vi "AdaptToInputs.vi"(3 "Term Types":T1, 4 "XRef":refnum<vi>, 5 "State In":T5) -> (0 "Reply":string[](array[string]), 2 "State Out":T5)   [LabVIEW 2012, in "Array Size and Index.xnode"]
uses:
  Array Size and Index.xnode
  State.ctl
  <vilib>/XNodeSupport/XNodeTermTypeIDPairs.ctl
  <vilib>/XNodeSupport/XNodeTermTypeIDPair.ctl
  <vilib>/XNodeSupport/XNodeType.ctl
  <vilib>/XNodeSupport/XNodeString.ctl
  <userlib>/_LAVAcr/Scripting Tools/XNode Support/Find term type by ID_type.vi
  <userlib>/_LAVAcr/Scripting Tools/XNode Support/XNode Support.lvlib
  <vilib>/XNodeSupport/NI_XNodeSupport.lvlib
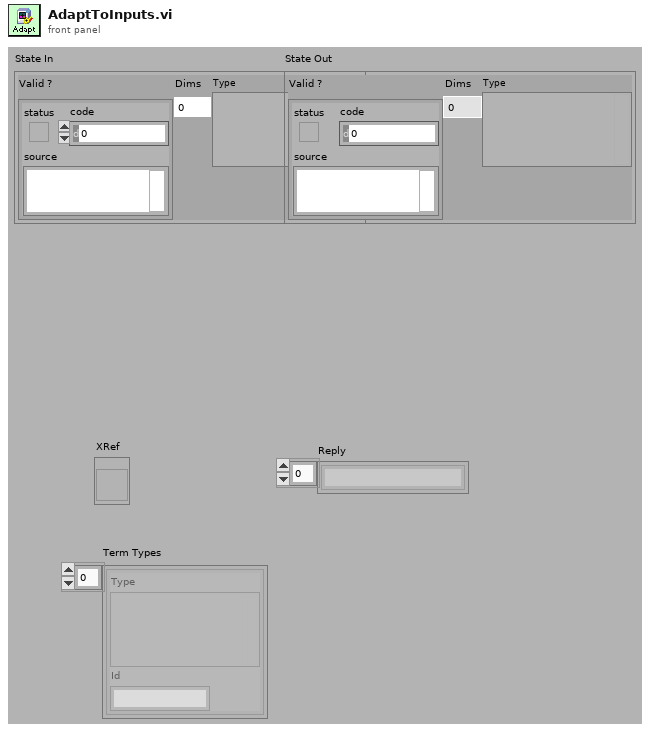
[diagram p1: front panel]
types:
  T1 = typedef "NI_XNodeSupport.lvlib/XNodeTermTypeIDPairs.ctl" = T2[]
  T2 = typedef "NI_XNodeSupport.lvlib/XNodeTermTypeIDPair.ctl" = cluster{"Type":T3, "Id":T4}
  T3 = typedef "NI_XNodeSupport.lvlib/XNodeType.ctl" = variant
  T4 = typedef "NI_XNodeSupport.lvlib/XNodeString.ctl" = string
  T5 = typedef "Array Size and Index.xnode/State.ctl" = cluster{"Valid ?":errorcluster, "Dims":i32, "Type":variant}
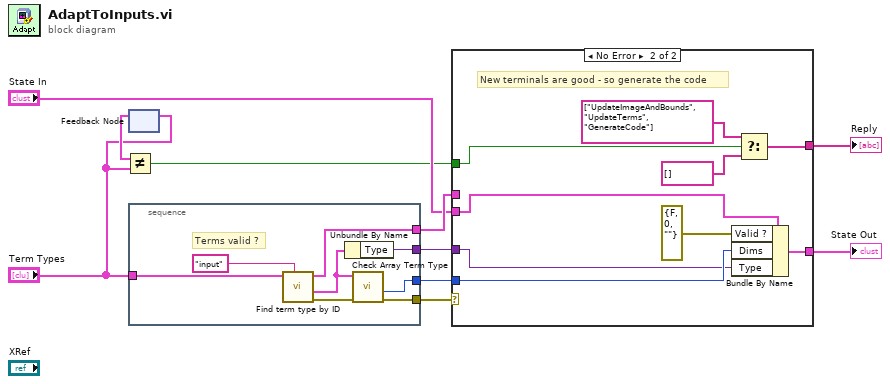
[diagram p0: block diagram]
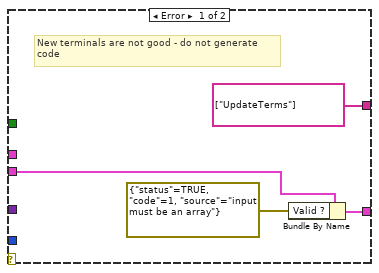
[diagram p2: hidden frame]
diagram:
  n1 = feedback-in #1("Term Types") -> ()
  n2 = feedback #1() -> (w3:T1)  [unwired: 1 out]
  n3 = Not Equal?(x=w3, y="Term Types") -> (x != y?=w1:bool)
  n4 = stacked-sequence {
    tunnel: "Term Types" -> [w18]
    tunnel: [w17] -> w9
    tunnel: [w14] -> w10
    tunnel: [w13] -> w5
    tunnel: [w11] -> w4
    frame #0 {
      # "Terms valid ?"
      n5 = call-poly <userlib>:"Find term type by ID.vi"("Search ID"="input", "Term Types"=w18) -> ("error out"=w15:errorcluster, "Term Type"=w12:T2, "Other Term Types"=w17:T2[])  [unwired: 1 in, 6 out]
      n6 = Unbundle By Name(w12) -> ("Type"=w11:T3)
      n7 = call <userlib>:"Check Array Term Type.vi"("error in (no error)"=w15, "Term Type"=w12) -> ("error out"=w14:errorcluster, "Array Dimensions"=w13:i32)  [unwired: 3 in, 5 out]
    }
  }
  n8 = case shown="No Error" w10 {
    tunnel: w9 -> [_ _]
    tunnel: "State In" -> [w22 w31]
    tunnel: [w20 w29] -> w7
    tunnel: [string[] ["UpdateTerms"] ("Reply") w25] -> w6
    tunnel: w5 -> [_ w28]
    tunnel: w4 -> [_ w27]
    tunnel: w1 -> [_ w23]
    frame Error {
      # "New terminals are not good - do not generate\ncode"
      n9 = Bundle By Name(cluster=w22, "Valid ?"=errorcluster {"status"=TRUE, "code"=1, "source"="input must be an array"}) -> (w20:T5)
    }
    frame No Error {
      # "New terminals are good - so generate the code"
      n10 = Bundle By Name(cluster=w31, "Valid ?"=errorcluster {"status"=FALSE, "code"=0, "source"=""}, "Dims"=w28, "Type"=w27) -> (w29:T5)
      n11 = Select(t=string[] ["UpdateImageAndBounds", "UpdateTerms", "GenerateCode"] ("Reply"), s=w23, f=string[] []) -> (s? t:f=w25:string[])
    }
  }
  "Reply" <- w6
  "State Out" <- w7
